vi "Shooter Gathering Velocity.vi"() -> ()   [LabVIEW 2012]
panel:
  in  "Shooter Gathering Velocity":dbl=-3000.0
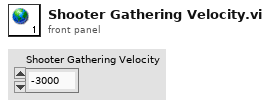
[diagram p1: front panel]
diagram:
